vi "User_Current_Write.vi"(8 "error in (no error)":errorcluster caption="错误输入（无错误）", 9 "Password":string, 10 "User_Right":string, 11 "Name":string) -> (0 "error out":errorcluster caption="错误输出")   [LabVIEW 2020]
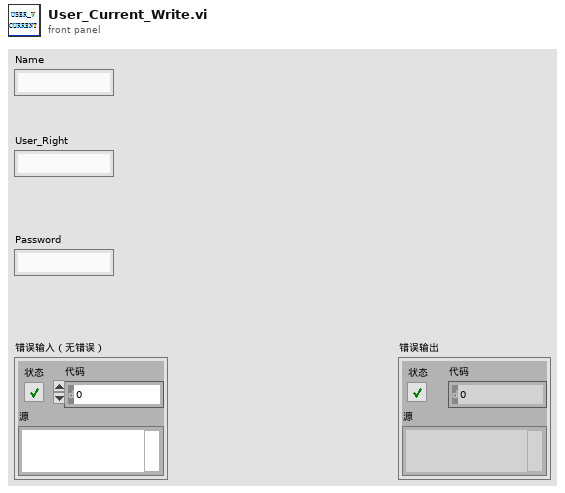
[diagram p1: front panel]
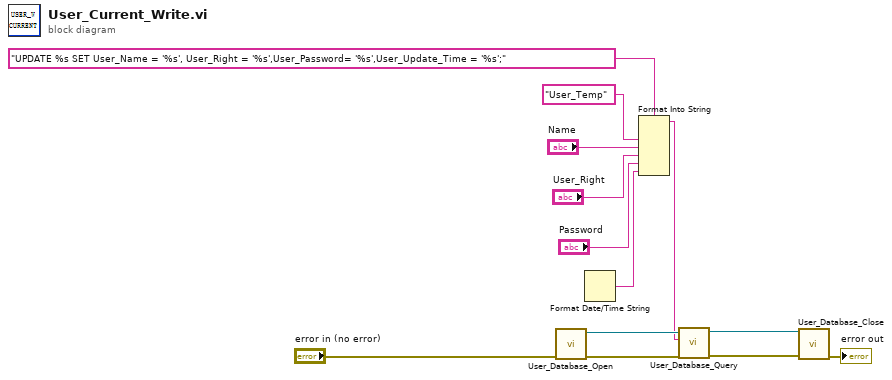
[diagram p0: block diagram]
diagram:
  n1 = call "User_Database_Open.vi"("error in (no error)"="error in (no error)") -> ("error out"=w11:errorcluster, "SQLite Connection"=w3:refnum<class "Connection.lvclass">)  [unwired: 9 in]
  n2 = Format Date/Time String() -> (date/time string=w1:string)  [unwired: 3 in]
  n3 = Format Into String(format string="UPDATE %s SET User_Name = '%s', User_Right = '%s',User_Password= '%s',User_Update_Time = '%s';", "User_Temp" ("table"), "Name", "User_Right", "Password", w1) -> (resulting string=w2:string)  [unwired: 2 in, 1 out]
  n4 = call "User_Database_Query.vi"("error in (no error)"=w11, "SQL query"=w2, "SQLite Connection in"=w3) -> ("error out"=w10:errorcluster, "SQLite Connection"=w9:refnum<class "Connection.lvclass">)  [unwired: 6 in, 1 out]
  n5 = call "User_Database_Close.vi"("error in (no error)"=w10, "SQLite Connection in"=w9) -> ("error out"=→"error out":errorcluster)  [unwired: 9 in]
